vi "CanData2Array.vi"(10 "Data":u8[](array[numeric]), 11 "COB ID":u32) -> (2 "Array":string[](array[string]))   [LabVIEW 2014]
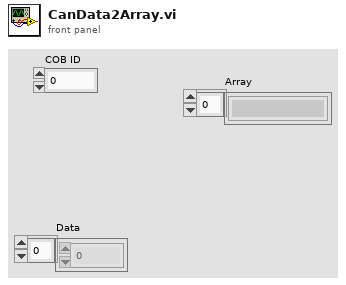
[diagram p1: front panel]
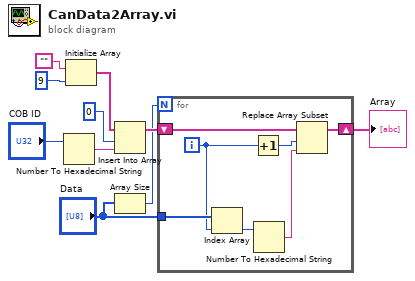
[diagram p0: block diagram]
diagram:
  n1 = Number To Hexadecimal String(2:"COB ID") -> (0:w6:string)  [unwired: 1 in]
  n2 = Initialize Array("" ("Element"), 9 ("Dimension")) -> (w5:string[])
  n3 = Insert Into Array(array=w5, index=0 ("Index"), new element=w6) -> (w2:string[])
  n4 = Array Size(array="Data") -> (size(s)=w1:i32)
  n5 = for {
    N: w1 -> [_]
    tunnel: "Data" -> [w15]
    shift-right: [w17] -> w3
    shift-left: w2 -> [w14]
    i -> [w12]
    n6 = Index Array(array=w15, index=w12) -> (element=w16:u8)
    n7 = Increment(x=w12) -> (x+1=w13:i32)
    n8 = Number To Hexadecimal String(2:w16) -> (0:w11:string)  [unwired: 1 in]
    n9 = Replace Array Subset(array=w14, new element=w11, index=w13) -> (w17:string[])
  }
  "Array" <- w3
